vi "Write ID.vi"(8 "error in (no error)":errorcluster, 10 "ID":string, 11 "Update Controller Data MSG in":refnum<class "Update Controller Data MSG.lvclass">) -> (0 "error out":errorcluster, 3 "Update Controller Data MSG out":refnum<class "Update Controller Data MSG.lvclass">)   [LabVIEW 2016, in "Controller.lvlib" / "Update Controller Data MSG.lvclass"]
uses:
  Update Controller Data MSG.lvclass
  Update Controller Data MSG.lvclass/Update Controller Data MSG.ctl
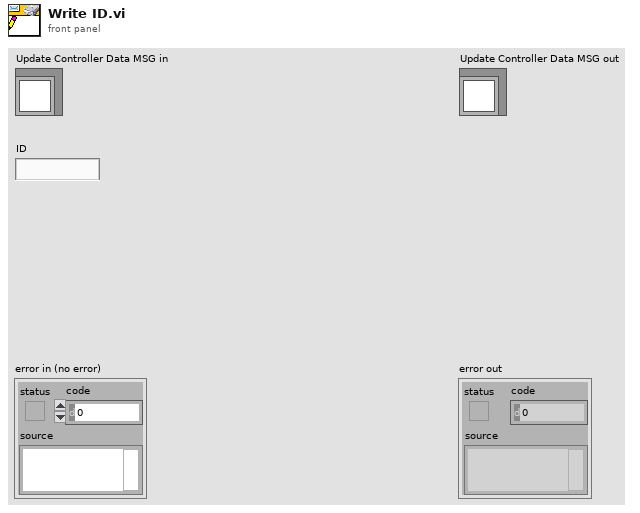
[diagram p1: front panel]
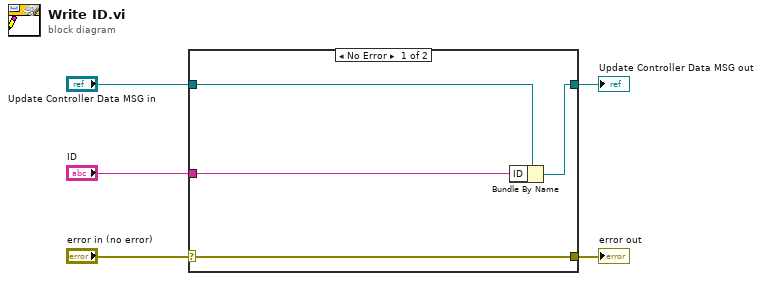
[diagram p0: block diagram]
diagram:
  n1 = case shown="No Error" "error in (no error)" {
    selector: "error in (no error)" -> [w9 w10]
    tunnel: [w9 w10] -> w4
    tunnel: [w7 w11] -> w2
    tunnel: "Update Controller Data MSG in" -> [w8 w11]
    tunnel: "ID" -> [w6 _]
    frame No Error {
      n2 = Bundle By Name(cluster=w8, "ID"=w6) -> (w7:refnum<class "Update Controller Data MSG.lvclass">)
    }
    frame Error {
    }
  }
  "error out" <- w4
  "Update Controller Data MSG out" <- w2
